vi "Motion Profiler.vi"(8 "From shift":T1, 10 "Current Location":dbl, 11 "Setpoint":dbl) -> (0 "To Shift":T1, 3 "Motion Profiler Setpoint output":dbl)   [LabVIEW 2014]
uses:
  TimeSegment.ctl
  TimeSegments.ctl
  Profiler Shift.ctl
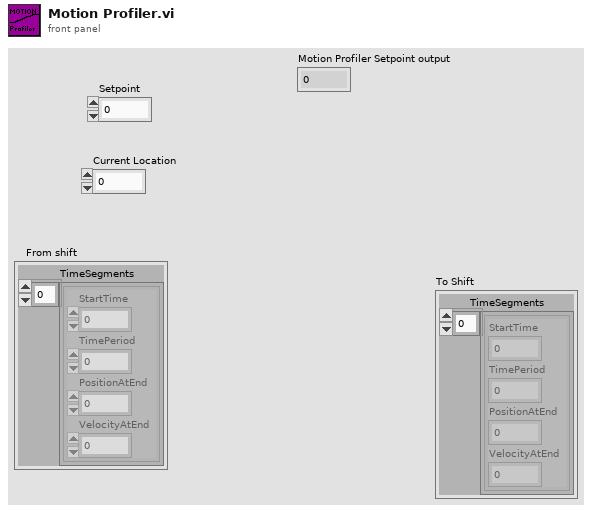
[diagram p1: front panel]
types:
  T1 = typedef "Profiler Shift.ctl" = cluster{"TimeSegments":T2}
  T2 = typedef "TimeSegments.ctl" = T3[]
  T3 = typedef "TimeSegment.ctl" = cluster{"StartTime":dbl, "TimePeriod":dbl, "PositionAtEnd":dbl, "VelocityAtEnd":dbl}
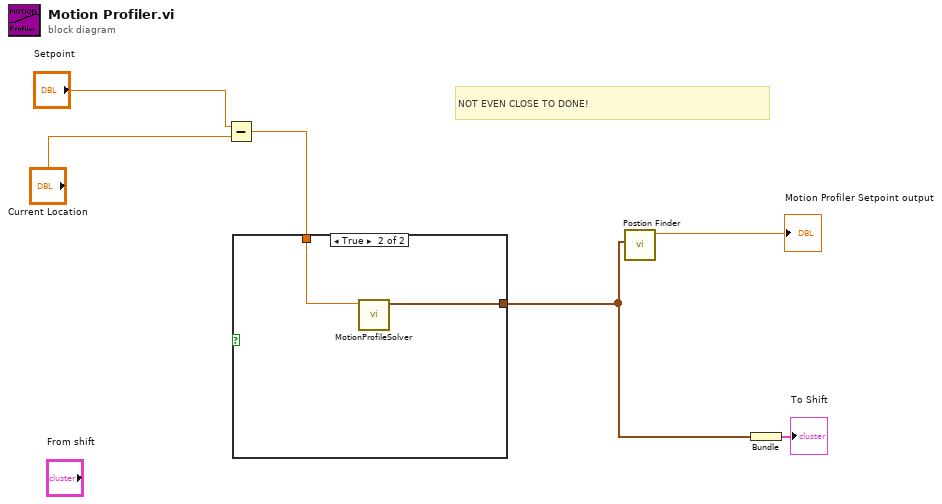
[diagram p0: block diagram]
diagram:
  # "NOT EVEN CLOSE TO DONE!"
  n1 = Subtract(x="Setpoint", y="Current Location") -> (x-y=w3:dbl)
  n2 = case shown="True" {
    selector: _ -> [_ _]
    tunnel: [_ w8] -> w2
    tunnel: w3 -> [_ w7]
    frame False {
    }
    frame True {
      n3 = call "MotionProfileSolver.vi"("Distance to go"=w7) -> ("TimeSegments"=w8:T2)  [unwired: 10 in]
    }
  }
  n4 = call "Postion Finder.vi"("TimeSegments"=w2) -> ("Motion Profiler Setpoint"=→"Motion Profiler Setpoint output":dbl)  [unwired: 10 in]
  n5 = Bundle("TimeSegments"=w2) -> (→"To Shift":cluster{"TimeSegments":T2})  [unwired: 1 in]
